vi "To Variant.vi"(8 "Error In":errorcluster, 11 "2D Flt":refnum<class "2D Flt.lvclass">) -> (0 "Error Out":errorcluster, 2 "Variant":variant)   [LabVIEW 2017, in "Tree API.lvlib" / "2D Flt.lvclass"]
doc: "Dynamic dispatch interface for conversion of Tree Data classes to variant LV data."
uses:
  2D Flt.lvclass
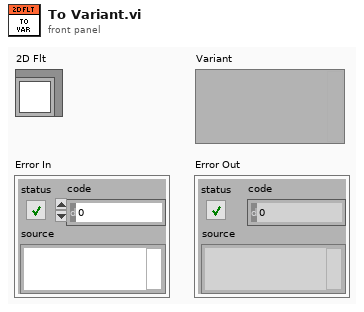
[diagram p1: front panel]
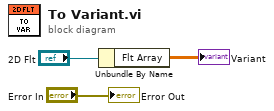
[diagram p0: block diagram]
diagram:
  n1 = Unbundle By Name("2D Flt") -> ("Flt Array"=→"Variant":dbl[][])
  "Error Out" <- "Error In"
